vi "XW_Psi_U_tweak_tester.vi"(2 "U2":dbl=10.0, 3 "U1":dbl=10.0, 4 "file path (dialog if empty)":path=path "E:/EnFlo Software/EnFlo Software/Anemometry/Anemometry Sub Vis/Calibration/Psi_U.txt") -> (0 "V":dbl, 1 "U":dbl)   [LabVIEW 2011]
panel:
  in  "Psi changes with U?":bool=TRUE
  in  "C2":dbl=0.5
  in  "C1":dbl=0.5
  in  "C0":dbl=1.0
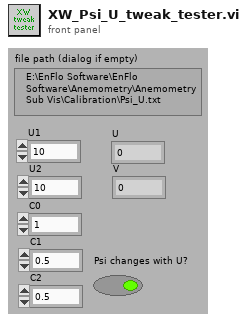
[diagram p1: front panel]
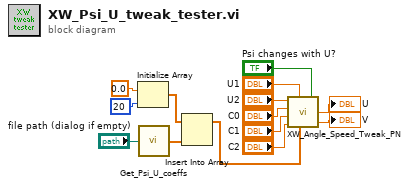
[diagram p0: block diagram]
diagram:
  n1 = Initialize Array(0.0 ("element"), 20 ("dimension size")) -> (w12:dbl[])
  n2 = call "Get_Psi_U_coeffs.vi"("file path (dialog if empty)"="file path (dialog if empty)") -> ("Coeffs to append"=w11:dbl[])
  n3 = Insert Into Array(array=w12, new element=w11) -> (w6:dbl[])  [unwired: 1 in]
  n4 = call "XW_Angle_Speed_Tweak_PN.vi"("U2"="U2", "U1"="U1", "C0"="C0", "C1"="C1", "Coeffs"=w6, "C2"="C2", "Psi changes with U?"="Psi changes with U?") -> ("U"=→"U":dbl, "V"=→"V":dbl)
